vi "Dispatch Read and Process UDP Messages.vi"(8 "error in":errorcluster, 9 "timeout (10 ms)":i32=10, 11 "UDP Conn ID":refnum<k16>) -> (0 "error out":errorcluster, 1 "Source Process":string, 2 "Sender Host":string, 3 "Message XML String":string, 4 "Message":T1, 5 "Receiver Process":string)   [LabVIEW 2014, in "AMC.lvlib"]
uses:
  AMC.lvlib
  Keyed Array/KeyedArray.ctl
  Keyed Array/Tools_KeyedArray.lvlib
  _SubVIs/TypeDefs/Message.ctl
panel:
  out "Message Length":i32
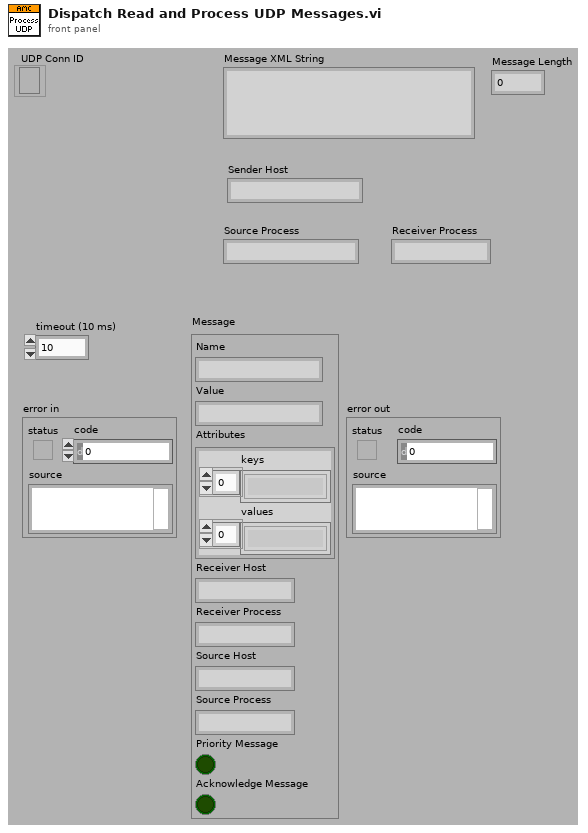
[diagram p1: front panel]
types:
  T1 = typedef "AMC.lvlib/Message.ctl" = cluster{"Name":string, "Value":string, "Attributes":T2, "Receiver Host":string, "Receiver Process":string, "Source Host":string, "Source Process":string, "Priority Message":bool, "Acknowledge Message":bool}
  T2 = typedef "Tools_KeyedArray.lvlib/KeyedArray.ctl" = cluster{"keys":string[], "values":string[]}
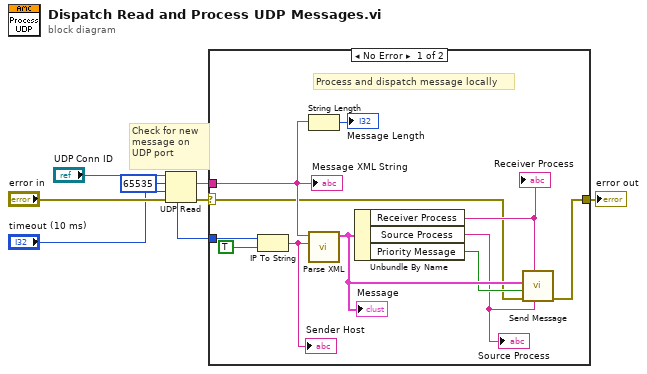
[diagram p0: block diagram]
diagram:
  # "Check for new\nmessage on\nUDP port"
  n1 = UDP Read(connection ID="UDP Conn ID", max size (548)=65535, timeout ms (25000)="timeout (10 ms)", 8:"error in") -> (data out=w4:string, error out=w7:errorcluster, 6:w6:u32)  [unwired: 2 out]
  n2 = case shown="No Error" w7 {
    selector: w7 -> [w11 w20]
    tunnel: w4 -> [w17 _]
    tunnel: w6 -> [w19 _]
    tunnel: [w10 w20] -> w2
    frame No Error {
      # "Process and dispatch message locally"
      n3 = IP To String(1:TRUE ("dot notation? (F)"), 2:w19) -> (0:w16:string)
      "Sender Host" <- w16
      n4 = String Length(string=w17) -> (length=→"Message Length":i32)
      n5 = call "Parse XML.vi"("Sender Host"=w16, "Message XML String"=w17) -> ("Message"=w15:T1)  [unwired: 9 out]
      "Message" <- w15
      n6 = Unbundle By Name(w15) -> ("Receiver Process"=w14:string, "Source Process"=w12:string, "Priority Message"=w13:bool)
      "Source Process" <- w12
      "Receiver Process" <- w14
      n7 = call "Send Message.vi"("Source Process"=w12, "Receiver Process"=w14, "error in (no error)"=w11, "Priority Message (F)"=w13, "Message"=w15) -> ("error out"=w10:errorcluster)  [unwired: 3 in, 3 out]
      "Message XML String" <- w17
    }
    frame Error {
    }
  }
  "error out" <- w2
